vi "dfd_NStage MRate Passband Ripple Modification.vi"(8 "error in (no error)":errorcluster, 9 "ripple specs":T1={"passband"=1.0, "stopband"=60.0, "dB/linear? (T: dB)"=TRUE}, 11 "#stages":i32=2) -> (0 "error out":errorcluster, 1 "ripple specs (dB)":T1={"passband"=0.05437453093312722, "stopband"=0.001, "dB/linear? (T: dB)"=FALSE})   [LabVIEW 2017, in "NI_DigFilterLicensed.lvlib"]
uses:
  <vilib>/addons/Digital Filter Design/NI_DigFilterLicensed.lvlib
  <vilib>/addons/Digital Filter Design/_Objects.llb/DFD Filter Ripple Specification (Design).ctl
  <vilib>/addons/Digital Filter Design/_Objects.llb/DFD Filter Frequence Specification (Design).ctl
  <vilib>/addons/Digital Filter Design/NI_DigFilter_Design.lvlib
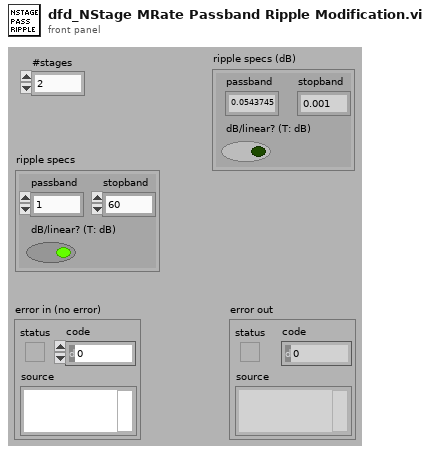
[diagram p1: front panel]
types:
  T1 = typedef "NI_DigFilterLicensed.lvlib/DFD Filter Ripple Specification (Design).ctl" = cluster{"passband":dbl, "stopband":dbl, "dB/linear? (T: dB)":bool}
  T2 = enum16{"Lowpass", "Highpass", "Bandpass", "Bandstop"}
  T3 = typedef "NI_DigFilterLicensed.lvlib/DFD Filter Frequence Specification (Design).ctl" = cluster{"fpass 1":dbl, "fstop 1":dbl, "fpass 2 ":dbl, "fstop 2":dbl}
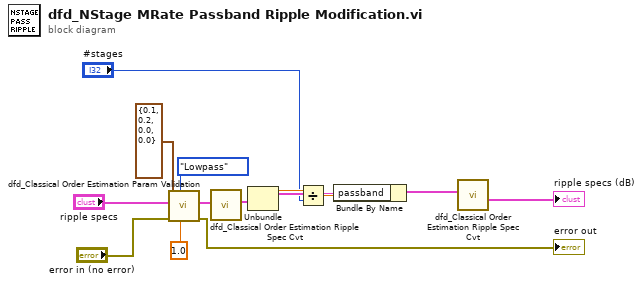
[diagram p0: block diagram]
diagram:
  n1 = call <vilib>:"dfd_Classical Order Estimation Param Validation.vi"("fs [Hz]"=1.0, "filter type"=T2."Lowpass", "error in (no error)"="error in (no error)", "ripple specs"="ripple specs", "freq specs [Hz]"=T3 {"fpass 1"=0.1, "fstop 1"=0.2, "fpass 2 "=0.0, "fstop 2"=0.0}) -> ("error out"=→"error out":errorcluster, "dup ripple specs"=w7:T1)  [unwired: 5 out]
  n2 = call <vilib>:"dfd_Classical Order Estimation Ripple Spec Cvt.vi"("ripple specs"=w7) -> ("ripple specs (linear)"=w12:T1)  [unwired: 10 out]
  n3 = Unbundle(w12) -> ("passband"=w10:dbl)  [unwired: 2 out]
  n4 = Divide(x=w10, y="#stages") -> (x/y=w13:dbl)
  n5 = Bundle By Name(cluster=w12, "passband"=w13) -> (w11:T1)
  n6 = call <vilib>:"dfd_Classical Order Estimation Ripple Spec Cvt.vi"("ripple specs"=w11) -> ("ripple specs (dB)"=→"ripple specs (dB)":T1)  [unwired: 10 out]
